vi "set Control State.vi"(10 "Control State":refnum<class "Control State.lvclass">, 11 "Ship in":refnum<class "Ship.lvclass">) -> (3 "Ship out":refnum<class "Ship.lvclass">)   [LabVIEW 2021, in "Ship.lvclass"]
uses:
  Ship.lvclass
  Control State/Control State.lvclass
  Ship.lvclass/Ship.ctl
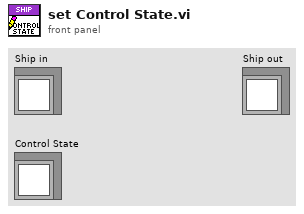
[diagram p1: front panel]
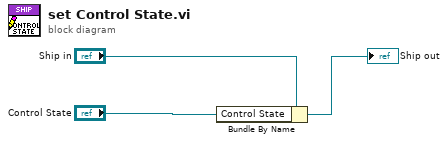
[diagram p0: block diagram]
diagram:
  n1 = Bundle By Name(cluster="Ship in", "Control State"="Control State") -> (→"Ship out":refnum<class "Ship.lvclass">)
